vi "NI5112.get bin data.vi"(0 "i ref in":refnum<vi>, 3 "ms timeout (100)":i32=100, 5 "error in (no error)":errorcluster) -> (14 "i ref out":refnum<vi>, 16 "Output Waveform":waveform(dbl)={"t0"=timestamp(0 s since 1904-01-01), "dt"=0.001, "Y"=array[1000 elements]}, 17 "timed out":bool, 19 "error out":errorcluster)   [LabVIEW 2014, in "NI5112.lvlib"]
uses:
  NI5112.lvlib
panel:
  in  "Case Constant\n(See Context Help) 4":bool
  in  "Case Constant\n(See Context Help) 3":bool
  in  "Case Constant\n(See Context Help) 2":bool
  in  "Case Constant\n(See Context Help)":bool
  out "real NI5112 data":dbl[](graph)
  out "discrData":i16[](graph)
  out "data to MM":i32[](graph)
  out "NI5112 data":i8[](graph)
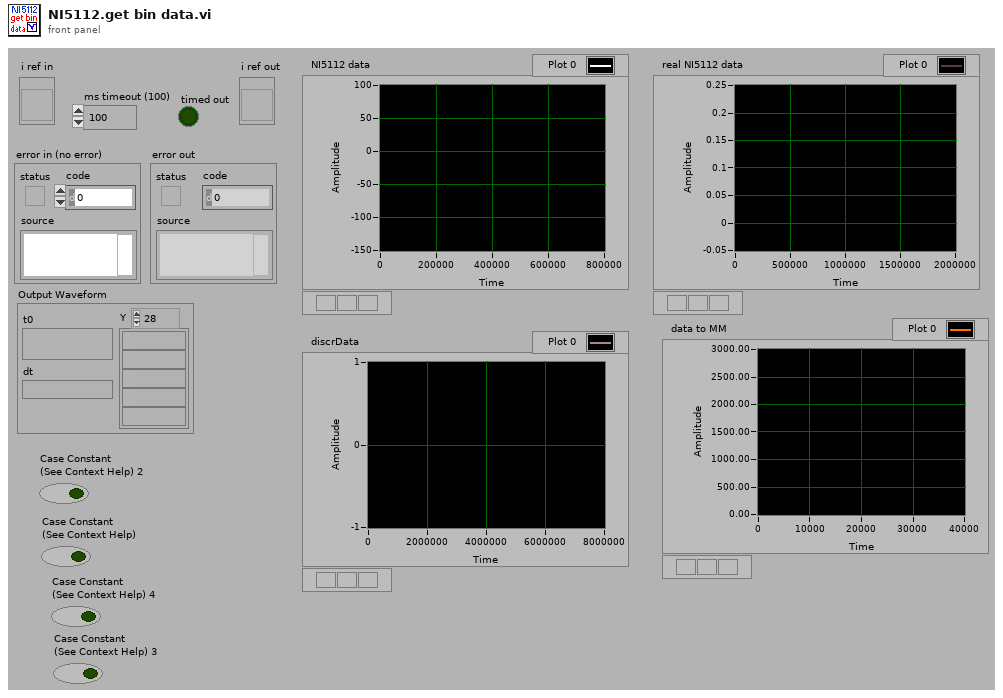
[diagram p1: front panel]
types:
  T1 = typedef "NI5112.lvlib/NI5112.i attribute.ctl" = cluster{"HWChannel":string, "instrument handle":refnum<k15>, "BinWidth":dbl, "vertical offset":dbl, "vertical range":dbl, "DataBPR":i32, "5112BPR":i32, "FullSpeed":bool, "discrLevel":dbl, "DoDiscr":bool, "VerCoupling":string}
  T2 = cluster{"actualSamples":i32, "absoluteInitialX":dbl, "relativeInitialX":dbl, "xIncrement":dbl, "offset":dbl, "gain":dbl, "reserved1":dbl, "reserved2":dbl}
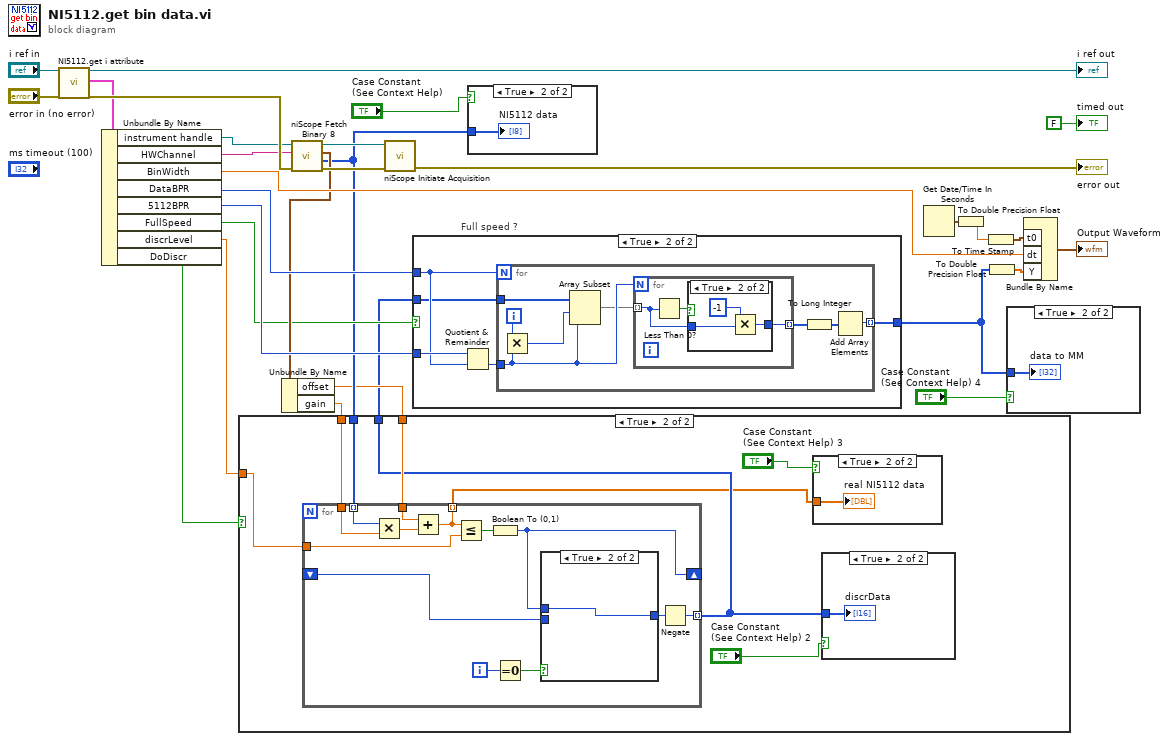
[diagram p0: block diagram]
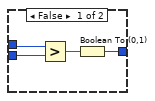
[diagram p5: hidden frame]
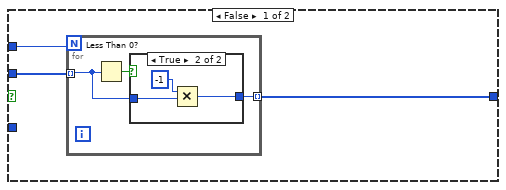
[diagram p8: hidden frame]
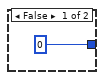
[diagram p9: hidden frame]
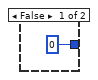
[diagram p10: hidden frame]
diagram:
  n1 = call "NI5112.get i attribute.vi"("i ref in"="i ref in", "error in (no error)"="error in (no error)") -> ("i ref out"=→"i ref out":refnum<vi>, "i attribute"=w27:T1, "error out"=w28:errorcluster)  [unwired: 15 in]
  n2 = Unbundle By Name(w27) -> ("instrument handle"=w26:refnum<k15>, "HWChannel"=w25:string, "BinWidth"=w16:dbl, "DataBPR"=w12:i32, "5112BPR"=w13:i32, "FullSpeed"=w7:bool, "discrLevel"=w3:dbl, "DoDiscr"=w2:bool)
  n3 = call <instrlib>:"niScope Fetch Binary 8.vi"("error in"=w28, "channels"=w25, "instrument handle"=w26) -> ("error out"=w15:errorcluster, "wfm"=w6:i8[], "wfm info"=w8:T2, "instrument handle out"=w18:refnum<k15>)  [unwired: 5 in]
  n4 = Unbundle By Name(w8) -> ("offset"=w4:dbl, "gain"=w5:dbl)
  n5 = case shown="True" w2 {
    tunnel: w6 -> [w31 w36]
    tunnel: w5 -> [_ w39]
    tunnel: w4 -> [_ w38]
    tunnel: w3 -> [_ w37]
    tunnel: [w31 w34] -> w1
    frame False {
    }
    frame True {
      n6 = for {
        tunnel: w36 -> [w54] mode=indexing
        tunnel: w39 -> [w53]
        tunnel: w38 -> [w52]
        tunnel: w37 -> [w50]
        shift-right: [w46] -> _
        shift-left: _ -> [w45]
        tunnel: [w43] -> w34 mode=indexing
        tunnel: [w42] -> w32 mode=indexing
        i -> [w47]
        n7 = Multiply(x=w54, y=w53) -> (x*y=w51:dbl)
        n8 = Add(x=w52, y=w51) -> (x+y=w42:dbl)
        n9 = Less Or Equal?(x=w42, y=w50) -> (x <= y?=w49:bool)
        n10 = Boolean To (0,1)(Boolean=w49) -> (0, 1=w46:i16)
        n11 = Equal To 0?(x=w47) -> (x = 0?=w48:bool)
        n12 = case shown="True" w48 {
          tunnel: w46 -> [w58 w59]
          tunnel: [w56 w59] -> w44
          tunnel: w45 -> [w55 _]
          frame False {
            n13 = Greater?(x=w58, y=w55) -> (0:w57:bool)
            n14 = Boolean To (0,1)(Boolean=w57) -> (0, 1=w56:i16)
          }
          frame True {
          }
        }
        n15 = Negate(x=w44) -> (-x=w43:i16)
      }
      n16 = case shown="True" "Case Constant\n(See Context Help) 3" {
        tunnel: w32 -> [_ w40]
        frame False {
        }
        frame True {
          "real NI5112 data" <- w40
        }
      }
      n17 = case shown="True" "Case Constant\n(See Context Help) 2" {
        tunnel: w34 -> [_ w41]
        frame False {
        }
        frame True {
          "discrData" <- w41
        }
      }
    }
  }
  n18 = call <instrlib>:"niScope Initiate Acquisition.vi"("instrument handle"=w18, "error in"=w15) -> ("error out"=→"error out":errorcluster)  [unwired: 12 in, 1 out]
  n19 = case "Full speed ?" shown="True" w7 {
    tunnel: [w61 w74] -> w9
    tunnel: w1 -> [w62 w70]
    tunnel: w13 -> [_ w73]
    tunnel: w12 -> [w60 w71]
    frame False {
      n20 = for {
        N: w60 -> [_]
        tunnel: w62 -> [w63] mode=indexing
        tunnel: [w64] -> w61 mode=indexing
        n21 = Less Than 0?(x=w63) -> (x < 0?=w65:bool)
        n22 = case shown="True" w65 {
          tunnel: [i16 0 w67] -> w64
          tunnel: w63 -> [_ w69]
          frame False {
          }
          frame True {
            n23 = Multiply(x=i16 -1, y=w69) -> (x*y=w67:i16)
          }
        }
      }
    }
    frame True {
      n24 = Quotient & Remainder(x=w73, y=w71) -> (floor(x/y)=w72:i32)  [unwired: 1 out]
      n25 = for {
        N: w71 -> [_]
        tunnel: w70 -> [w82]
        tunnel: [w76] -> w74 mode=indexing
        tunnel: w72 -> [w78]
        i -> [w81]
        n26 = Multiply(x=w81, y=w78) -> (x*y=w80:i32)
        n27 = Array Subset(array=w82, index=w80, length=w78) -> (w77:i16[])
        n28 = for {
          N: w78 -> [_]
          tunnel: w77 -> [w84] mode=indexing
          tunnel: [w83] -> w75 mode=indexing
          n29 = Less Than 0?(x=w84) -> (x < 0?=w85:bool)
          n30 = case shown="True" w85 {
            tunnel: [i16 0 w87] -> w83
            tunnel: w84 -> [_ w89]
            frame False {
            }
            frame True {
              n31 = Multiply(x=-1, y=w89) -> (x*y=w87:i32)
            }
          }
        }
        n32 = To Long Integer(number=w75) -> (32bit integer=w79:i32[])
        n33 = Add Array Elements(numeric array=w79) -> (sum=w76:i32)
      }
    }
  }
  n34 = case shown="True" "Case Constant\n(See Context Help)" {
    tunnel: w6 -> [_ w90]
    frame False {
    }
    frame True {
      "NI5112 data" <- w90
    }
  }
  n35 = Get Date/Time In Seconds() -> (seconds since 1Jan1904=w23:timestamp)
  n36 = To Double Precision Float(number=w23) -> (double precision float=w24:dbl)
  n37 = To Time Stamp(1:w24) -> (0:w22:timestamp)
  n38 = To Double Precision Float(number=w9) -> (double precision float=w19:dbl[])
  n39 = case shown="True" "Case Constant\n(See Context Help) 4" {
    tunnel: w9 -> [_ w91]
    frame False {
    }
    frame True {
      "data to MM" <- w91
    }
  }
  n40 = Bundle By Name("t0"=w22, "dt"=w16, "Y"=w19) -> (→"Output Waveform":waveform(dbl))  [unwired: 1 in]
  "timed out" <- FALSE ("timed out")
